vi "Create DO Channel.vi"(6 "index":i32, 8 "error in":errorcluster, 9 "default value":bool, 10 "name":string, 11 "DO channel in":refnum<class "DO Channel.lvclass">) -> (0 "error out":errorcluster, 3 "DO channel out":refnum<class "DO Channel.lvclass">)   [LabVIEW 2017, in "Scan Engine Scripting.lvlib" / "DO Channel.lvclass"]
doc: "Creates an instance of a digital output channel."
uses:
  DO Channel.lvclass
  Channel/Type.ctl
  Channel/Channel.lvclass
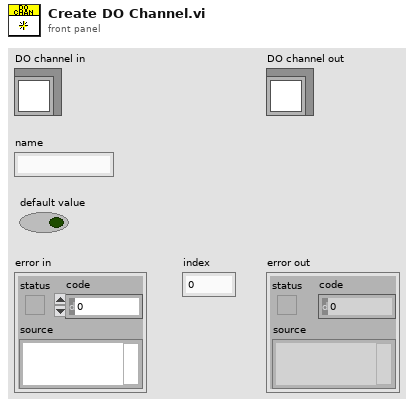
[diagram p1: front panel]
types:
  T1 = typedef "Scan Engine Scripting.lvlib/Channel.lvclass/Type.ctl" = enum16{"Input", "Output"}
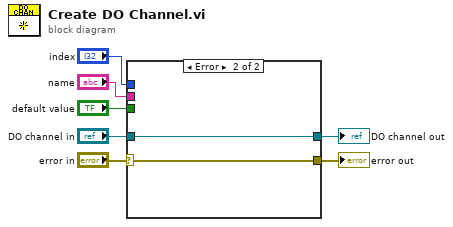
[diagram p0: block diagram]
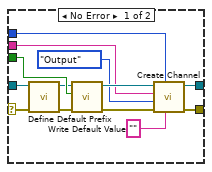
[diagram p2: hidden frame]
diagram:
  n1 = case shown="Error" "error in" {
    selector: "error in" -> [w8 w22]
    tunnel: "name" -> [w16 _]
    tunnel: "default value" -> [w15 _]
    tunnel: [w14 w22] -> w5
    tunnel: [w13 w21] -> w4
    tunnel: "index" -> [w12 _]
    tunnel: "DO channel in" -> [w11 w21]
    frame No Error {
      n2 = call-dynamic "Define Default Prefix.vi"("error in (no error)"=w8, "DO Channel in"=w11) -> ("error out"=w10:errorcluster, "DO Channel out"=w9:refnum<class "DO Channel.lvclass">)  [unwired: 8 in]
      n3 = call-dynamic "Write Default Value.vi"("error in"=w10, "default value"=w15, "digital channel in"=w9) -> ("error out"=w20:errorcluster, "digital channel out"=w19:refnum<class "DO Channel.lvclass">)  [unwired: 7 in]
      n4 = call-dynamic "Create Channel.vi"("units"="", "index"=w12, "error in"=w20, "type"=Type."Output", "name"=w16, "channel in"=w19) -> ("error out"=w14:errorcluster, "channel out"=w13:refnum<class "DO Channel.lvclass">)  [unwired: 4 in]
    }
    frame Error {
    }
  }
  "error out" <- w5
  "DO channel out" <- w4
